vi "filter_luz.vi"(11 "Datos Leídos Luz 3":string[](array[string])=["0", "0", "2", "8", "6", "0", "0", "1", "D", "A", "0", "0", "1", "A", "2", "0", "0", "1", "8", "C", "0", "0", "1", "7", "4", "0", "0", "1", "6", "A", "0", "0", "1", "8", "E", "0", "0", "1", "9", "1", "0", "0", "1", "7", "2", "0", "0", "1", "6", "B", "0", "0", "1", "8", "3", "0", "0", "1", "6", "9", "0", "0", "1", "9", "C", "0", "0", "1", "7", "3", "0", "0", "1", "8", "7", "0", "0", "1", "8", "E", "0", "0", "1", "A", "9", "0", "0", "1", "8", "7", "0", "0", "1", "6", "3", "0", "0", "1", "8", "7", "0", "0", "1", "7", "8", "0", "0", "1", "A", "0", "0", "0", "1", "8", "6", "0", "0", "1", "8", "4", "0", "0", "1", "A", "D", "0", "0", "1", "9", "2", "0", "0", "1", "A", "8", "0", "0", "1", "9", "6", "0", "0", "1", "6", "D", "0", "0", "1", "6", "5", "0", "0", "1", "8", "A", "0", "0", "1", "6", "7", "0", "0", "1", "A", "6", "0", "0", "1", "6", "9", "0", "0", "1", "8", "9", "0", "0", "1", "8", "D", "0", "0", "1", "7", "5", "0", "0", "1", "7", "6", "0", "0", "1", "7", "4", "0", "0", "1", "7", "9", "0", "0", "1", "9", "9", "0", "0", "1", "8", "1", "0", "0", "1", "8", "E", "0", "0", "1", "7", "F", "0", "0", "1", "7", "6", "0", "0", "1", "9", "6", "0", "0", "1", "8", "5", "0", "0", "1", "9", "B", "0", "0", "1", "7", "6", "0", "0", "1", "7", "D", "0", "0", "1", "7", "0", "0", "0", "1", "8", "8", "0", "0", "1", "8", "0", "0", "0", "1", "A", "7", "0", "0", "1", "9", "F", "0", "0", "1", "9", "1", "0", "0", "1", "7", "5", "0", "0", "1", "7", "4", "0", "0", "1", "7", "2", "0", "0", "1", "6", "9", "0", "0", "1", "9", "4", "0", "0", "1", "8", "2", "0", "0", "1", "8", "9", "0", "0", "1", "9", "B", "0", "0", "1", "5", "F", "0", "0", "1", "9", "3", "0", "0", "1", "5", "D", "0", "0", "1", "9", "5", "0", "0", "1", "5", "6", "0", "0", "1", "7", "5", "0", "0", "1", "9", "E", "0", "0", "1", "7", "4", "0", "0", "1", "6", "F", "0", "0", "1", "8", "9", "0", "0", "1", "A", "D", "0", "0", "1", "8", "9", "0", "0", "1", "7", "D", "0", "0", "1", "6", "A", "0", "0", "1", "8", "C", "0", "0", "1", "6", "6", "0", "0", "1", "6", "F", "0", "0", "1", "7", "7", "0", "0", "1", "9", "6", "0", "0", "1", "8", "4", "0", "0", "1", "8", "E", "0", "0", "1", "7", "9", "0", "0", "1", "8", "7", "0", "0", "1", "7", "C", "0", "0", "1", "A", "A", "0", "0", "1", "7", "7", "0", "0", "1", "6", "8", "0", "0", "1", "8", "6", "0", "0", "1", "8", "3", "0", "0", "1", "6", "4", "0", "0", "1", "9", "8", "0", "0", "1", "8", "4", "0", "0", "1", "8", "4", "0", "0", "1", "8", "0", "0", "0", "1", "9", "0", "0", "0", "1", "6", "C", "0", "0", "1", "9", "0", "0", "0", "1", "8", "D", "0", "0", "1", "7", "D", "0", "0", "1", "8", "3", "0", "0", "1", "9", "6", "0", "0", "1", "6", "8", "0", "0", "1", "9", "5", "0", "0", "1", "9", "0", "0", "0", "1", "7", "D", "0", "0", "1", "9", "0", "0", "0", "1", "9", "6", "0", "0", "1", "6", "F", "0", "0", "1", "8", "9", "0", "0", "1", "8", "D", "0", "0", "1", "8", "B", "0", "0", "1", "8", "7", "0", "0", "1", "7", "1", "0", "0", "1", "8", "2", "0", "0", "1", "8", "0", "0", "0", "1", "5", "5", "0", "0", "1", "9", "D", "0", "0", "1", "8", "5", "0", "0", "1", "5", "A", "0", "0", "1", "8", "E", "0", "0", "1", "9", "1", "0", "0", "1", "9", "0", "0", "0", "1", "B", "C", "0", "0", "1", "6", "A", "0", "0", "1", "8", "1", "0", "0", "1", "8", "4", "0", "0", "1", "8", "C", "0", "0", "1", "8", "8", "0", "0", "1", "6", "A", "0", "0", "1", "8", "B", "0", "0", "1", "6", "D", "0", "0", "1", "9", "B", "0", "0", "1", "8", "9", "0", "0", "1", "7", "A", "0", "0", "1", "7", "D", "0", "0", "1", "6", "F", "0", "0", "1", "8", "7", "0", "0", "1", "5", "0", "0", "0", "1", "7", "7", "0", "0", "1", "8", "5", "0", "0", "1", "9", "1", "0", "0", "1", "8", "9", "0", "0", "1", "8", "1", "0", "0", "1", "8", "6", "0", "0", "1", "8", "3", "0", "0", "1", "A", "6", "0", "0", "1", "7", "C", "0", "0", "1", "7", "F", "0", "0", "1", "7", "9", "0", "0", "1", "7", "3", "0", "0", "1", "8", "4", "0", "0", "1", "6", "4", "0", "0", "1", "7", "B", "0", "0", "1", "8", "5", "0", "0", "1", "6", "9", "0", "0", "1", "7", "0", "0", "0", "1", "6", "B", "0", "0", "1", "9", "6", "0", "0", "1", "7", "7", "0", "0", "1", "9", "0", "0", "0", "1", "A", "3", "0", "0", "1", "9", "4", "0", "0", "1", "7", "9", "0", "0", "1", "8", "3", "0", "0", "1", "7", "A", "0", "0", "1", "9", "B", "0", "0", "1", "6", "B", "0", "0", "1", "9", "2", "0", "0", "1", "9", "4", "0", "0", "1", "8", "E", "0", "0", "1", "7", "5", "0", "0", "1", "8", "3", "0", "0", "1", "9", "2", "0", "0", "1", "8", "C", "0", "0", "1", "6", "C", "0", "0", "1", "8", "8", "0", "0", "1", "6", "4", "0", "0", "1", "A", "E", "0", "0", "1", "6", "5", "0", "0", "1", "8", "2", "0", "0", "1", "5", "C", "0", "0", "1", "7", "E", "0", "0", "1", "8", "B", "0", "0", "1", "8", "4", "0", "0", "1", "6", "B", "0", "0", "1", "B", "4", "0", "0", "1", "9", "1", "0", "0", "1", "7", "D", "0", "0", "1", "7", "F", "0", "0", "1", "8", "D", "0", "0", "1", "8", "6", "0", "0", "1", "8", "A", "0", "0", "1", "9", "0", "0", "0", "1", "6", "A", "0", "0", "1", "8", "D", "0", "0", "1", "7", "6", "0", "0", "1", "A", "4", "0", "0", "1", "8", "A", "0", "0", "1", "7", "3", "0", "0", "1", "8", "2", "0", "0", "1", "8", "D", "0", "0", "1", "9", "9", "0", "0", "1", "5", "D", "0", "0", "1", "8", "2", "0", "0", "1", "7", "9", "0", "0", "1", "9", "3", "0", "0", "1", "6", "F", "0", "0", "1", "8", "A", "0", "0", "1", "8", "2", "0", "0", "1", "9", "0", "0", "0", "1", "8", "8", "0", "0", "1", "7", "F", "0", "0", "1", "8", "5", "0", "0", "1", "8", "4", "0", "0", "1", "8", "5", "0", "0", "1", "B", "B", "0", "0", "1", "A", "8", "0", "0", "1", "5", "D", "0", "0", "1", "7", "4", "0", "0", "1", "9", "0", "0", "0", "1", "7", "5", "0", "0", "1", "9", "D", "0", "0", "1", "9", "A", "0", "0", "1", "7", "0", "0", "0", "1", "8", "1", "0", "0", "1", "8", "5", "0", "0", "1", "8", "3", "0", "0", "1", "9", "A", "0", "0", "1", "6", "4", "0", "0", "1", "7", "6", "0", "0", "1", "7", "9", "0", "0", "1", "A", "4", "0", "0", "1", "8", "9", "0", "0", "1", "6", "3", "0", "0", "1", "9", "2", "0", "0", "1", "6", "B", "0", "0", "1", "7", "4", "0", "0", "1", "9", "3", "0", "0", "1", "9", "F", "0", "0", "1", "7", "B", "0", "0", "1", "8", "2", "0", "0", "1", "8", "6", "0", "0", "1", "7", "A", "0", "0", "1", "9", "8", "0", "0", "1", "6", "1", "0", "0", "1", "8", "8", "0", "0", "1", "A", "A", "0", "0", "1", "7", "C", "0", "0", "1", "8", "1", "0", "0", "1", "7", "9", "0", "0", "1", "5", "5", "0", "0", "1", "7", "8", "0", "0", "1", "7", "1", "0", "0", "1", "8", "4", "0", "0", "1", "8", "3", "0", "0", "1", "8", "4", "0", "0", "1", "7", "3", "0", "0", "1", "6", "F", "0", "0", "1", "6", "C", "0", "0", "1", "9", "5", "0", "0", "1", "6", "E", "0", "0", "1", "7", "D", "0", "0", "1", "9", "5", "0", "0", "1", "8", "3", "0", "0", "1", "7", "0", "0", "0", "1", "8", "3", "0", "0", "1", "6", "5", "0", "0", "1", "7", "F", "0", "0", "1", "6", "5", "\u0004"]) -> (3 "Curva de luz":cluster{"Ramp Pattern":dbl[], u32[]}(graph))   [LabVIEW 2021]
uses:
  <vilib>/Analysis/1siggen.llb/Ramp Pattern by Delta.vi
  <vilib>/Analysis/NI_AALBase.lvlib
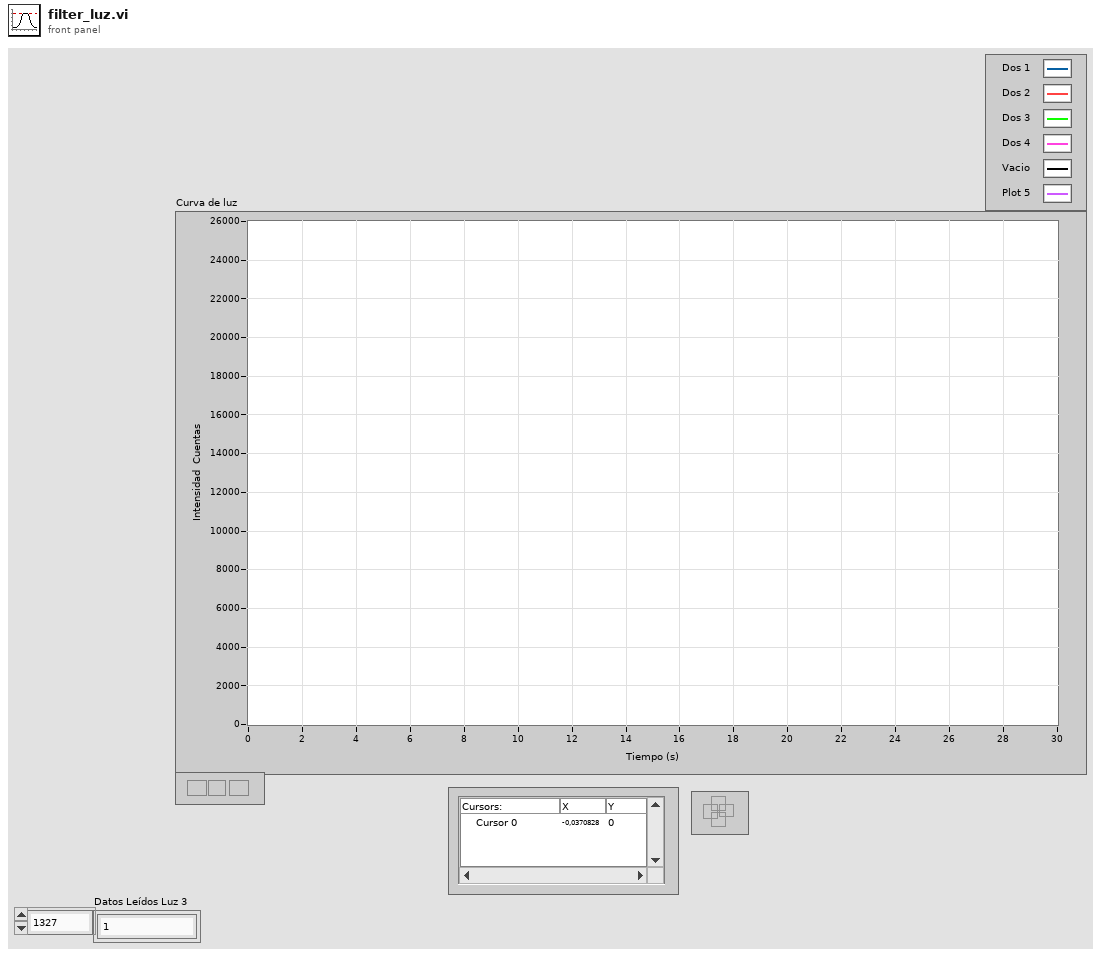
[diagram p1: front panel]
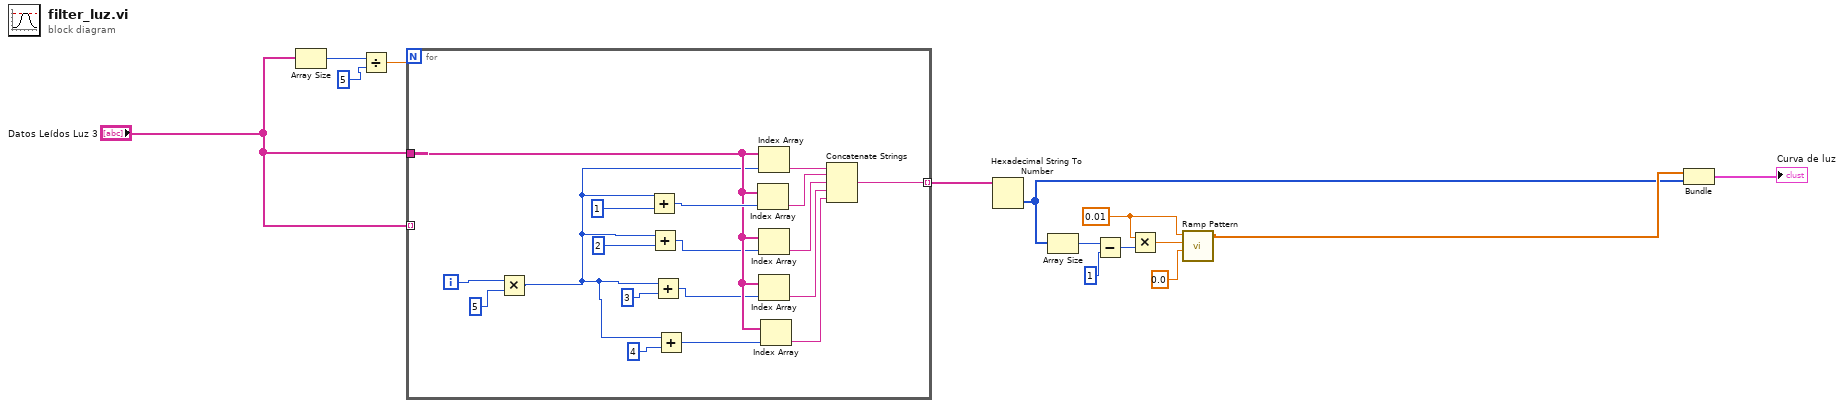
[diagram p0: block diagram]
diagram:
  w8 = 0.01 ("delta")
  n1 = Array Size(array="Datos Leídos Luz 3") -> (size(s)=w9:i32)
  n2 = Divide(x=w9, y=5) -> (x/y=w11:dbl)
  n3 = for {
    N: w11 -> [_]
    tunnel: "Datos Leídos Luz 3" -> [_] mode=indexing
    tunnel: "Datos Leídos Luz 3" -> [w23]
    tunnel: [w29] -> w12 mode=indexing
    i -> [w25]
    n4 = Multiply(x=w25, y=5) -> (x*y=w17:i32)
    n5 = Add(x=w17, y=1) -> (x+y=w26:i32)
    n6 = Add(x=w17, y=2) -> (x+y=w22:i32)
    n7 = Add(x=w17, y=3) -> (x+y=w21:i32)
    n8 = Add(x=w17, y=4) -> (x+y=w19:i32)
    n9 = Index Array(array=w23, index=w26) -> (element=w31:string)
    n10 = Index Array(array=w23, index=w17) -> (element=w32:string)
    n11 = Index Array(array=w23, index=w22) -> (element=w30:string)
    n12 = Index Array(array=w23, index=w21) -> (element=w16:string)
    n13 = Index Array(array=w23, index=w19) -> (element=w15:string)
    n14 = Concatenate Strings(w32, w31, w30, w16, w15) -> (w29:string)
  }
  n15 = Hexadecimal String To Number(string=w12) -> (number=w2:u32[])  [unwired: 2 in, 1 out]
  n16 = Array Size(array=w2) -> (size(s)=w6:i32)
  n17 = Subtract(x=w6, y=1) -> (x-y=w4:i32)
  n18 = Multiply(x=w8, y=w4) -> (x*y=w7:dbl)
  n19 = call-poly <vilib>:"Ramp Pattern.vi"("start"=0.0, "end"=w7, "delta"=w8) -> ("Ramp Pattern"=w14:dbl[])  [unwired: 6 in, 2 out]
  n20 = Bundle("Ramp Pattern"=w14, w2) -> (→"Curva de luz":cluster{"Ramp Pattern":dbl[], u32[]})  [unwired: 1 in]
